vi "CPSControlling.vi"() -> ()   [LabVIEW 2017]
uses:
  classes/DataHandlerMYiTOPS.lvclass
panel:
  in  "Monitoring":T1 {"Meter" scale=0.0..20.0}
  out "appended array":string[](array[string])
  out "element":string
  out "Control-Matrix-Overview 2":i32(listbox)=-1
  in  "Controlling":T2={"LED 1"=FALSE, "Stop Client App"=FALSE, "LED 2"=FALSE, "Drive Motor"=FALSE, "Direcion Moter"=FALSE, "Steps"=512} {"Steps" min=1 step=1}
  in  "Cyber-physical Objects":i32(listbox)
  in  "Stop":bool
  out "Control-Matrix-Overview":i32(listbox)=-1
  # "Hard Key:"
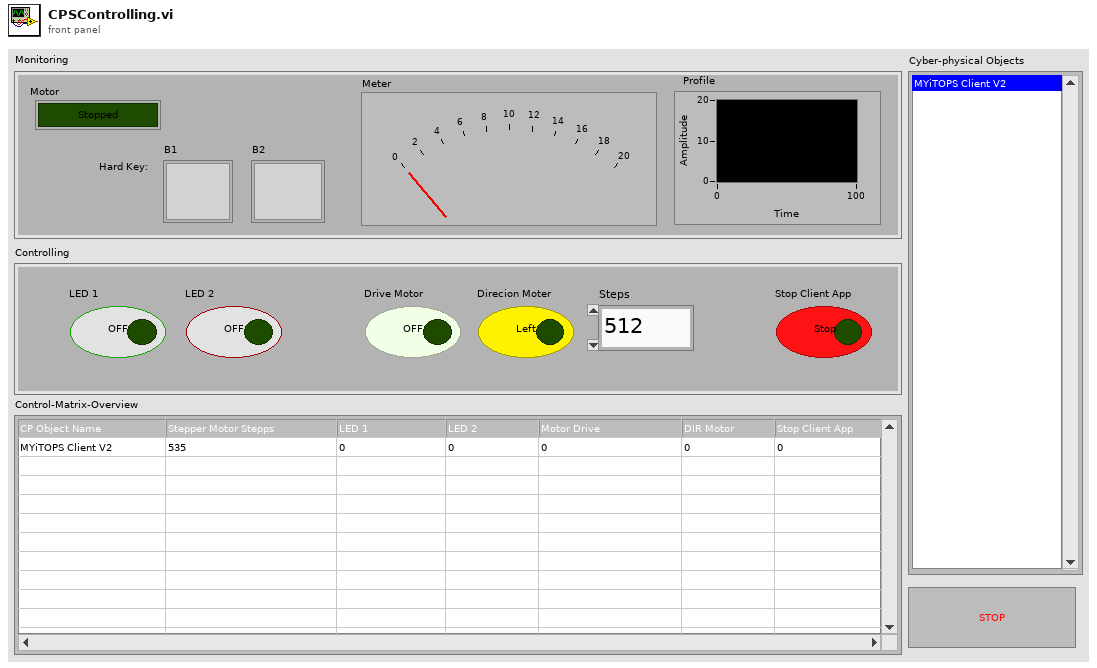
[diagram p1: front panel]
types:
  T1 = cluster{"Meter":i8, "Profile":dbl, "B2":bool, "B1":bool, "Motor":bool}
  T2 = cluster{"LED 1":bool, "Stop Client App":bool, "LED 2":bool, "Drive Motor":bool, "Direcion Moter":bool, "Steps":u64}
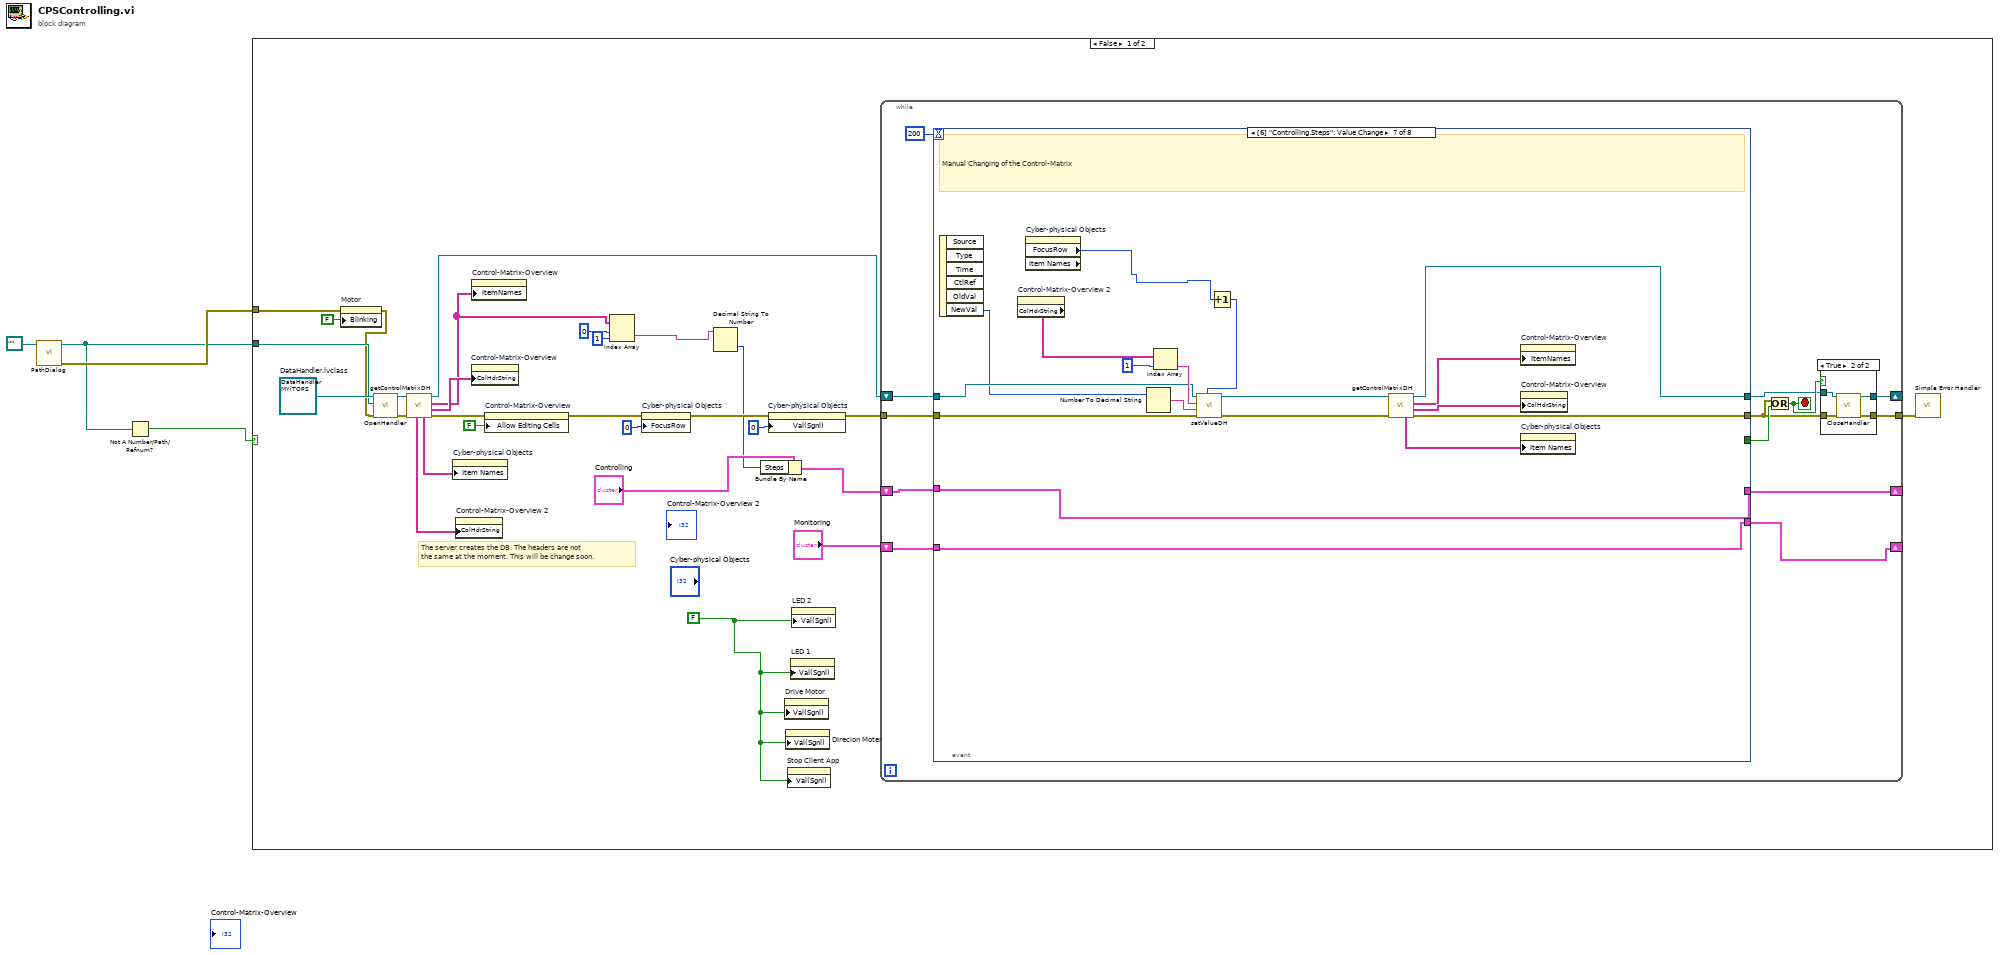
[diagram p0: block diagram]
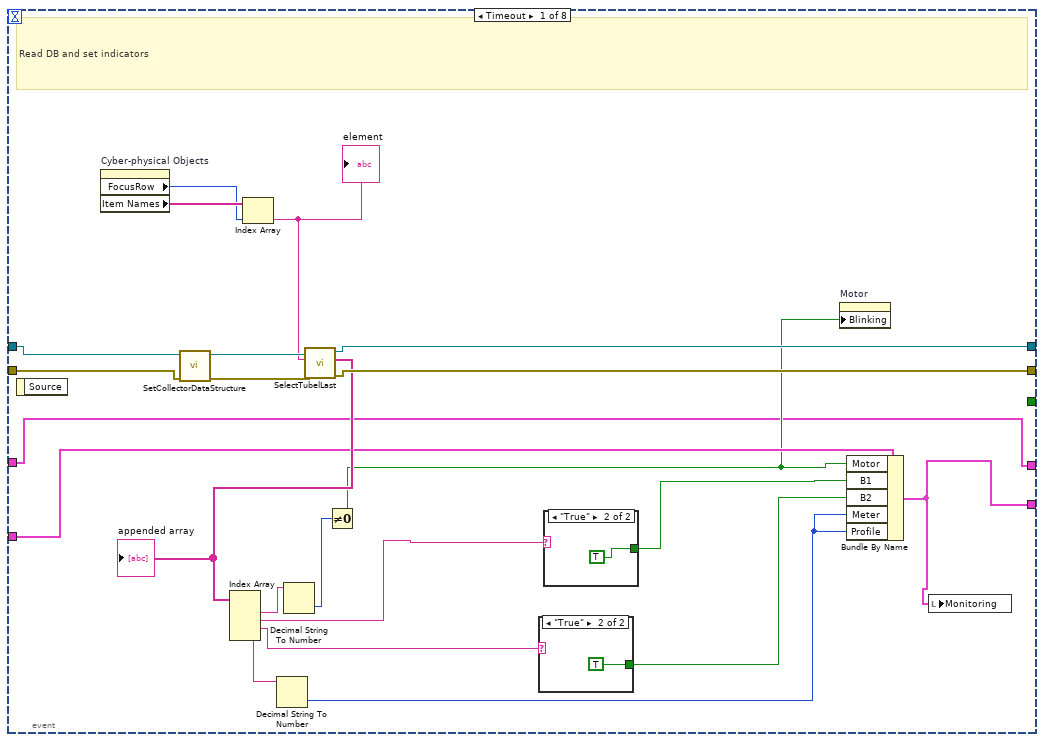
[diagram p3: hidden frame]
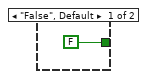
[diagram p4: hidden frame]
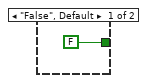
[diagram p5: hidden frame]
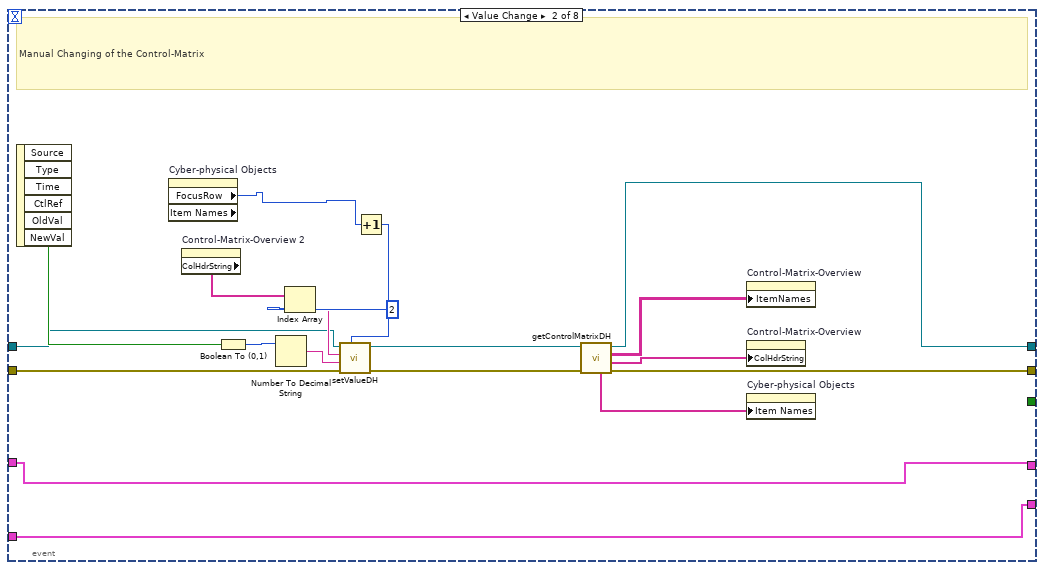
[diagram p6: hidden frame]
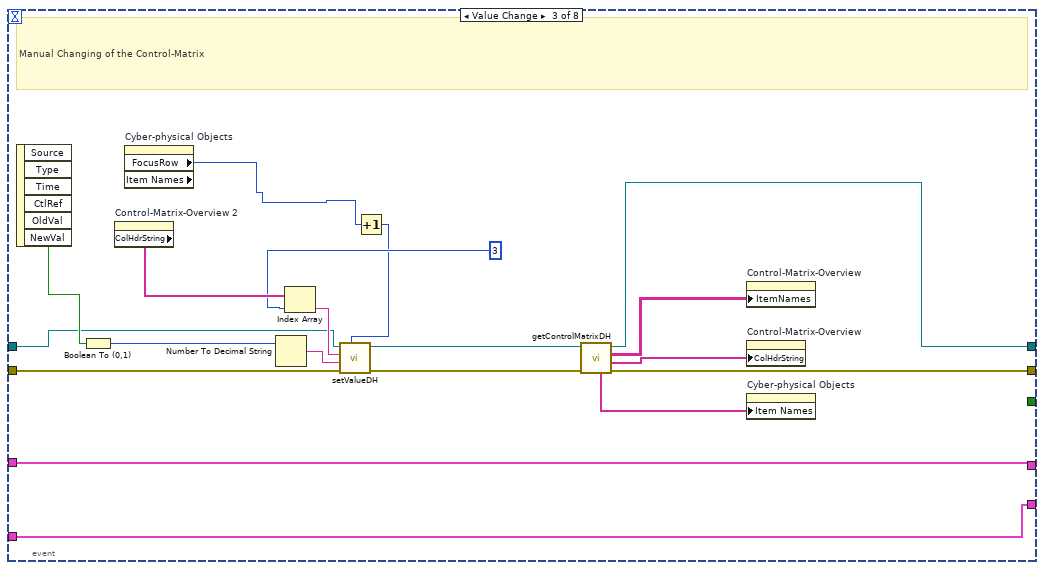
[diagram p7: hidden frame]
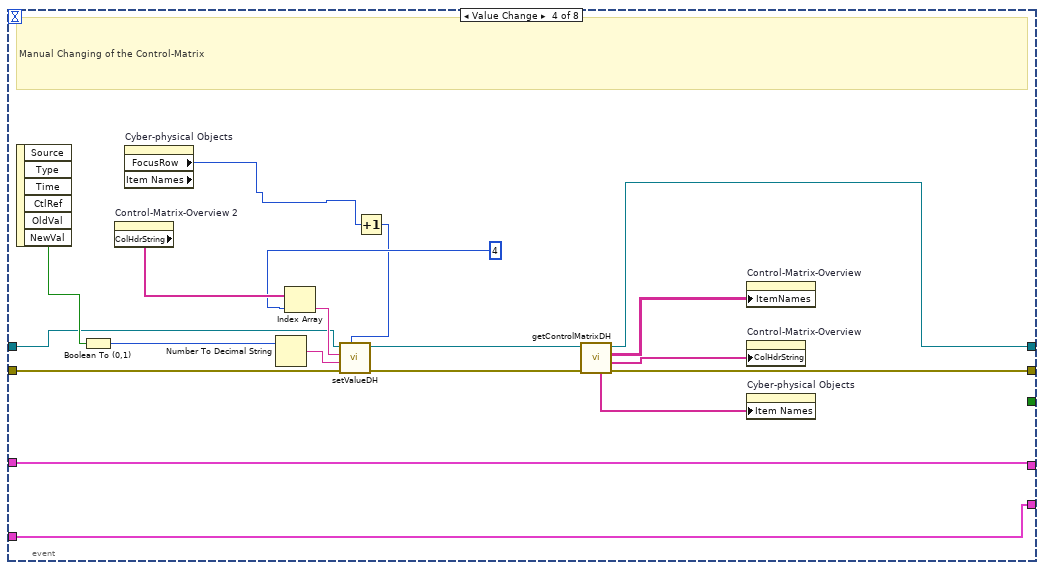
[diagram p8: hidden frame]
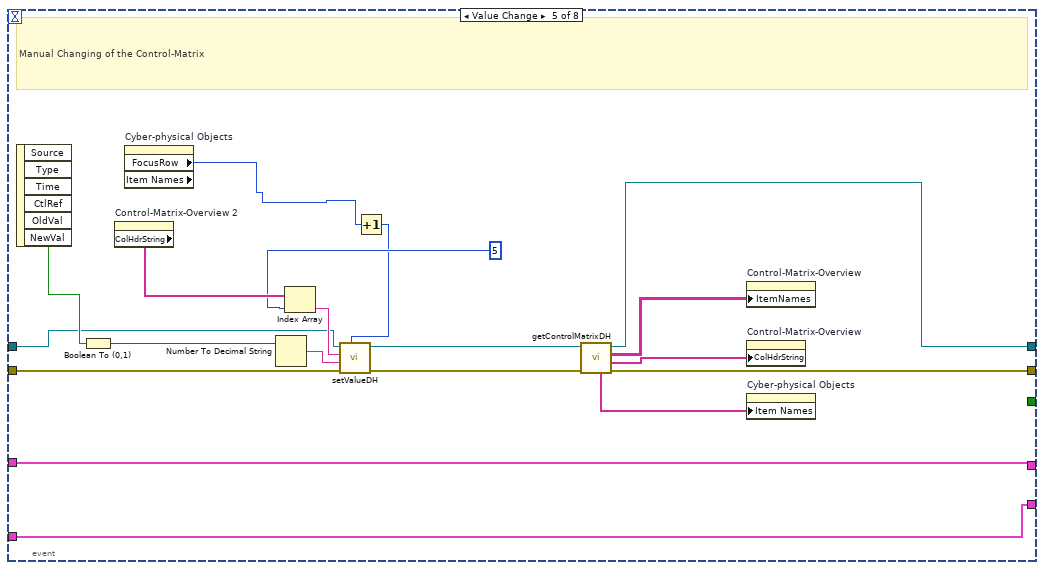
[diagram p9: hidden frame]
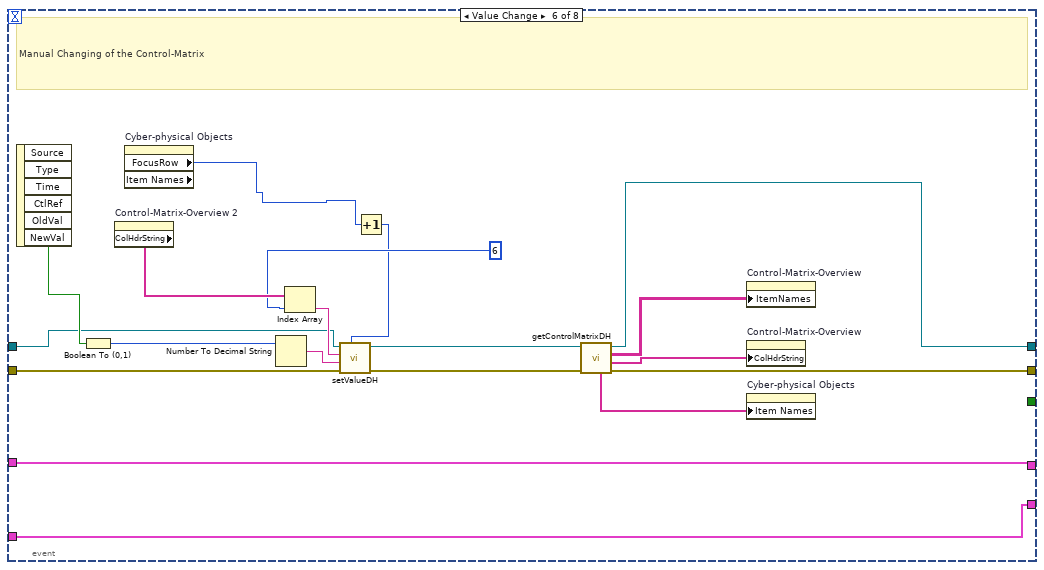
[diagram p10: hidden frame]
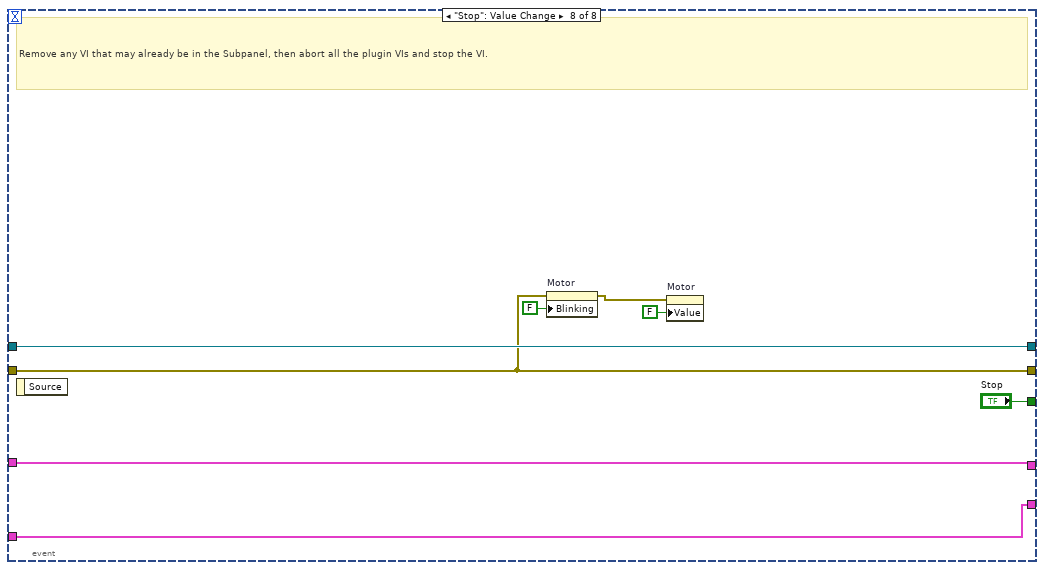
[diagram p11: hidden frame]
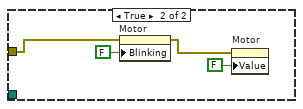
[diagram p12: hidden frame]
diagram:
  n1 = call "PathDialog.vi"("Path to Data Base in"=path "" ("Path to Data Base")) -> ("error out"=w3:errorcluster, "Path to Data Base out"=w2:path)  [unwired: 9 in]
  n2 = Not A Number/Path/Refnum?(number/path/refnum=w2) -> (NaN/Path/Refnum?=w1:bool)
  n3 = case shown="False" w1 {
    tunnel: w2 -> [w17 _]
    tunnel: w3 -> [w14 w201]
    frame False {
      w15 = FALSE ("Value")
      w28 = refnum<class "DataHandlerMYiTOPS.lvclass"> refnum  # DataHandler.lvclass
      # "The server creates the DB. The headers are not \nthe same at the moment. This will be change soon."
      n4 = property on="Motor" class="Bool (strict)"(error in=w14, "Blinking"=FALSE) -> (error out=w13:errorcluster)  [unwired: 1 in, 1 out]
      n5 = call-dynamic "OpenHandler.vi"("error in (no error)"=w13, "path to db monitoring"=w17, "DataHandling in"=w28) -> ("error out"=w27:errorcluster, "DataHandling out"=w26:refnum<class "DataHandlerMYiTOPS.lvclass">)  [unwired: 7 in]
      n6 = call-dynamic "getControlMatrixDH.vi"("error in (no error)"=w27, "DataHandler in"=w26) -> ("error out"=w24:errorcluster, "List of ColHads"=w23:string[], "Array"=w10:string[][], "DataHandler out"=w19:refnum<class "DataHandlerMYiTOPS.lvclass">, "Field Elements"=w25:string[], "List of ColHads 2"=w18:string[])  [unwired: 4 in]
      n7 = property on="Cyber-physical Objects" class="LstBox (strict)"("Item Names"=w25) -> ()  [unwired: 2 in, 2 out]
      n8 = property on="Control-Matrix-Overview 2" class="MCListbox (strict)"("ColHdrString"=w18) -> ()  [unwired: 2 in, 2 out]
      n9 = property on="Control-Matrix-Overview" class="MCListbox (strict)"("ColHdrString"=w23) -> ()  [unwired: 2 in, 2 out]
      n10 = property on="Control-Matrix-Overview" class="MCListbox (strict)"("ItemNames"=w10) -> ()  [unwired: 2 in, 2 out]
      n11 = property on="Control-Matrix-Overview" class="MCListbox (strict)"(error in=w24, "Allow Editing Cells"=FALSE) -> (error out=w20:errorcluster)  [unwired: 1 in, 1 out]
      n12 = Index Array(array=w10, index (row)=0 ("index"), index (col)=1 ("disabled index (col)")) -> (element=w6:string)
      n13 = property on="Cyber-physical Objects" class="LstBox (strict)"(error in=w20, "FocusRow"=0 ("Focus Row")) -> (error out=w21:errorcluster)  [unwired: 1 in, 1 out]
      n14 = Decimal String To Number(string=w6) -> (number=w5:i32)  [unwired: 2 in, 1 out]
      n15 = Bundle By Name(cluster="Controlling", "Steps"=w5) -> (w7:T2)
      n16 = property on="Cyber-physical Objects" class="ListBox (strict)"(error in=w21, "Val(Sgnl)"=u16 0 ("Value (Signaling)")) -> (error out=w32:errorcluster)  [unwired: 1 in, 1 out]
      n17 = property on="Drive Motor" class="Bool (strict)"("Val(Sgnl)"=w15) -> ()  [unwired: 2 in, 2 out]
      n18 = property on="Direcion Moter" class="Bool (strict)"("Val(Sgnl)"=w15) -> ()  [unwired: 2 in, 2 out]
      n19 = property on="Stop Client App" class="Bool (strict)"("Val(Sgnl)"=w15) -> ()  [unwired: 2 in, 2 out]
      n20 = property on="LED 1" class="Bool (strict)"("Val(Sgnl)"=w15) -> ()  [unwired: 2 in, 2 out]
      n21 = property on="LED 2" class="Bool (strict)"("Val(Sgnl)"=w15) -> ()  [unwired: 2 in, 2 out]
      n22 = while {
        tunnel: w32 -> [w44]
        tunnel: [w39] -> w30
        shift-right: [w37] -> _
        shift-left: w19 -> [w42]
        shift-right: [w33] -> _
        shift-left: w7 -> [w36]
        shift-right: [w34] -> _
        shift-left: "Monitoring" -> [w35]
        stop <- w41 stop-if-true
        n23 = event shown="[6] \"Controlling.Steps\": Value Change" {
          selector: _ -> [_ _ _ _ _ _ _ _]
          dyn-events: _ -> [_ _ _ _ _ _ _ _]
          timeout: 200 -> [_ _ _ _ _ _ _ _]
          tunnel: [_ _ _ _ _ _ _ "Stop"] -> w45
          tunnel: [w66 w94 w111 w130 w149 w168 w186 w193] -> w40
          tunnel: w44 -> [w68 w96 w115 w134 w153 w172 w190 w193]
          tunnel: w42 -> [w71 w85 w102 w121 w140 w159 w179 w197]
          tunnel: [w69 w86 w103 w122 w141 w160 w180 w197] -> w38
          tunnel: w36 -> [w52 w82 w98 w117 w136 w155 w173 w196]
          tunnel: [w52 w82 w98 w117 w136 w155 w173 w196] -> w33
          tunnel: w35 -> [w56 w81 w97 w116 w135 w154 w175 w195]
          tunnel: [w55 w81 w97 w116 w135 w154 w175 w195] -> w34
          event Timeout {
            # "Read DB and set indicators"
            n24 = event-data() -> ()  [unwired: 1 in, 1 out]
            n25 = property on="Cyber-physical Objects" class="LstBox (strict)"() -> ("FocusRow"=w72:i32, "Item Names"=w73:string[])  [unwired: 2 in, 2 out]
            n26 = call-dynamic "SetCollectorDataStructure.vi"("error in (no error)"=w68, "DataHandler in"=w71) -> ("error out"=w67:errorcluster, "DataHandler out"=w70:refnum<class "DataHandlerMYiTOPS.lvclass">)  [unwired: 8 in]
            n27 = Index Array(array=w73, index=w72) -> (element=w65:string)
            "element" <- w65
            n28 = call-dynamic "SelectTubelLast.vi"("error in (no error)"=w67, "Unique Object Identifier"=w65, "DataHandler in"=w70) -> ("error out"=w66:errorcluster, "appended array"=w64:string[], "DataHandler out"=w69:refnum<class "DataHandlerMYiTOPS.lvclass">)  [unwired: 6 in]
            "appended array" <- w64
            n29 = Index Array(array=w64) -> (element #1=w63:string, element #2=w62:string, element #3=w61:string, element #4=w60:string)  [unwired: 4 in]
            n30 = Decimal String To Number(string=w60) -> (number=w59:i32)  [unwired: 2 in, 1 out]
            n31 = Decimal String To Number(string=w63) -> (number=w54:i32)  [unwired: 2 in, 1 out]
            n32 = Not Equal To 0?(x=w54) -> (x != 0?=w53:bool)
            n33 = case shown="\"True\"" w61 {
              tunnel: [FALSE TRUE] -> w58
              frame "False", Default {
              }
              frame "True" {
              }
            }
            n34 = case shown="\"True\"" w62 {
              tunnel: [FALSE TRUE] -> w57
              frame "False", Default {
              }
              frame "True" {
              }
            }
            n35 = property on="Motor" class="Bool (strict)"("Blinking"=w53) -> ()  [unwired: 2 in, 2 out]
            n36 = Bundle By Name(cluster=w56, "Motor"=w53, "B1"=w57, "B2"=w58, "Meter"=w59, "Profile"=w59) -> (w55:T1)
            n37 = local write "Monitoring"(w55) -> ()
          }
          event "Controlling.LED 1": Value Change {
            # "Manual Changing of the Control-Matrix"
            n38 = event-data() -> ("NewVal"=w89:bool)  [unwired: 1 in, 5 out]
            n39 = property on="Cyber-physical Objects" class="LstBox (strict)" props=["FocusRow", "Item Names"]() -> ("FocusRow"=w84:i32)  [unwired: 2 in, 3 out]
            n40 = property on="Control-Matrix-Overview 2" class="MCListbox (strict)"() -> ("ColHdrString"=w92:string[])  [unwired: 2 in, 2 out]
            n41 = Boolean To (0,1)(Boolean=w89) -> (0, 1=w88:i16)
            n42 = Number To Decimal String(number=w88) -> (decimal integer string=w93:string)  [unwired: 1 in]
            n43 = Index Array(array=w92, index=2) -> (element=w90:string)
            n44 = Increment(x=w84) -> (x+1=w83:i32)
            n45 = call-dynamic "setValueDH.vi"("Focus"=w83, "error in (no error)"=w96, "Value"=w93, "ItemName"=w90, "DataHandler in"=w85) -> ("error out"=w95:errorcluster, "DataHandler out"=w87:refnum<class "DataHandlerMYiTOPS.lvclass">)  [unwired: 5 in]
            n46 = call-dynamic "getControlMatrixDH.vi"("error in (no error)"=w95, "DataHandler in"=w87) -> ("error out"=w94:errorcluster, "List of ColHads"=w79:string[], "Array"=w78:string[][], "DataHandler out"=w86:refnum<class "DataHandlerMYiTOPS.lvclass">, "Field Elements"=w80:string[])  [unwired: 4 in, 1 out]
            n47 = property on="Control-Matrix-Overview" class="MCListbox (strict)"("ItemNames"=w78) -> ()  [unwired: 2 in, 2 out]
            n48 = property on="Control-Matrix-Overview" class="MCListbox (strict)"("ColHdrString"=w79) -> ()  [unwired: 2 in, 2 out]
            n49 = property on="Cyber-physical Objects" class="LstBox (strict)"("Item Names"=w80) -> ()  [unwired: 2 in, 2 out]
          }
          event "Controlling.LED 2": Value Change {
            # "Manual Changing of the Control-Matrix"
            n50 = event-data() -> ("NewVal"=w106:bool)  [unwired: 1 in, 5 out]
            n51 = Boolean To (0,1)(Boolean=w106) -> (0, 1=w105:i16)
            n52 = property on="Control-Matrix-Overview 2" class="MCListbox (strict)"() -> ("ColHdrString"=w109:string[])  [unwired: 2 in, 2 out]
            n53 = property on="Cyber-physical Objects" class="LstBox (strict)" props=["FocusRow", "Item Names"]() -> ("FocusRow"=w100:i32)  [unwired: 2 in, 3 out]
            n54 = Number To Decimal String(number=w105) -> (decimal integer string=w110:string)  [unwired: 1 in]
            n55 = Index Array(array=w109, index=3) -> (element=w107:string)
            n56 = Increment(x=w100) -> (x+1=w99:i32)
            n57 = call-dynamic "setValueDH.vi"("Focus"=w99, "error in (no error)"=w115, "Value"=w110, "ItemName"=w107, "DataHandler in"=w102) -> ("error out"=w112:errorcluster, "DataHandler out"=w104:refnum<class "DataHandlerMYiTOPS.lvclass">)  [unwired: 5 in]
            n58 = call-dynamic "getControlMatrixDH.vi"("error in (no error)"=w112, "DataHandler in"=w104) -> ("error out"=w111:errorcluster, "List of ColHads"=w113:string[], "Array"=w101:string[][], "DataHandler out"=w103:refnum<class "DataHandlerMYiTOPS.lvclass">, "Field Elements"=w114:string[])  [unwired: 4 in, 1 out]
            n59 = property on="Control-Matrix-Overview" class="MCListbox (strict)"("ItemNames"=w101) -> ()  [unwired: 2 in, 2 out]
            n60 = property on="Control-Matrix-Overview" class="MCListbox (strict)"("ColHdrString"=w113) -> ()  [unwired: 2 in, 2 out]
            n61 = property on="Cyber-physical Objects" class="LstBox (strict)"("Item Names"=w114) -> ()  [unwired: 2 in, 2 out]
          }
          event "Controlling.Drive Motor": Value Change {
            # "Manual Changing of the Control-Matrix"
            n62 = event-data() -> ("NewVal"=w125:bool)  [unwired: 1 in, 5 out]
            n63 = Boolean To (0,1)(Boolean=w125) -> (0, 1=w124:i16)
            n64 = property on="Control-Matrix-Overview 2" class="MCListbox (strict)"() -> ("ColHdrString"=w128:string[])  [unwired: 2 in, 2 out]
            n65 = property on="Cyber-physical Objects" class="LstBox (strict)" props=["FocusRow", "Item Names"]() -> ("FocusRow"=w119:i32)  [unwired: 2 in, 3 out]
            n66 = Number To Decimal String(number=w124) -> (decimal integer string=w129:string)  [unwired: 1 in]
            n67 = Index Array(array=w128, index=4) -> (element=w126:string)
            n68 = Increment(x=w119) -> (x+1=w118:i32)
            n69 = call-dynamic "setValueDH.vi"("Focus"=w118, "error in (no error)"=w134, "Value"=w129, "ItemName"=w126, "DataHandler in"=w121) -> ("error out"=w131:errorcluster, "DataHandler out"=w123:refnum<class "DataHandlerMYiTOPS.lvclass">)  [unwired: 5 in]
            n70 = call-dynamic "getControlMatrixDH.vi"("error in (no error)"=w131, "DataHandler in"=w123) -> ("error out"=w130:errorcluster, "List of ColHads"=w132:string[], "Array"=w120:string[][], "DataHandler out"=w122:refnum<class "DataHandlerMYiTOPS.lvclass">, "Field Elements"=w133:string[])  [unwired: 4 in, 1 out]
            n71 = property on="Control-Matrix-Overview" class="MCListbox (strict)"("ItemNames"=w120) -> ()  [unwired: 2 in, 2 out]
            n72 = property on="Control-Matrix-Overview" class="MCListbox (strict)"("ColHdrString"=w132) -> ()  [unwired: 2 in, 2 out]
            n73 = property on="Cyber-physical Objects" class="LstBox (strict)"("Item Names"=w133) -> ()  [unwired: 2 in, 2 out]
          }
          event "Controlling.Direcion Moter": Value Change {
            # "Manual Changing of the Control-Matrix"
            n74 = event-data() -> ("NewVal"=w144:bool)  [unwired: 1 in, 5 out]
            n75 = Boolean To (0,1)(Boolean=w144) -> (0, 1=w143:i16)
            n76 = property on="Control-Matrix-Overview 2" class="MCListbox (strict)"() -> ("ColHdrString"=w147:string[])  [unwired: 2 in, 2 out]
            n77 = property on="Cyber-physical Objects" class="LstBox (strict)" props=["FocusRow", "Item Names"]() -> ("FocusRow"=w138:i32)  [unwired: 2 in, 3 out]
            n78 = Number To Decimal String(number=w143) -> (decimal integer string=w148:string)  [unwired: 1 in]
            n79 = Index Array(array=w147, index=5) -> (element=w145:string)
            n80 = Increment(x=w138) -> (x+1=w137:i32)
            n81 = call-dynamic "setValueDH.vi"("Focus"=w137, "error in (no error)"=w153, "Value"=w148, "ItemName"=w145, "DataHandler in"=w140) -> ("error out"=w150:errorcluster, "DataHandler out"=w142:refnum<class "DataHandlerMYiTOPS.lvclass">)  [unwired: 5 in]
            n82 = call-dynamic "getControlMatrixDH.vi"("error in (no error)"=w150, "DataHandler in"=w142) -> ("error out"=w149:errorcluster, "List of ColHads"=w151:string[], "Array"=w139:string[][], "DataHandler out"=w141:refnum<class "DataHandlerMYiTOPS.lvclass">, "Field Elements"=w152:string[])  [unwired: 4 in, 1 out]
            n83 = property on="Control-Matrix-Overview" class="MCListbox (strict)"("ItemNames"=w139) -> ()  [unwired: 2 in, 2 out]
            n84 = property on="Control-Matrix-Overview" class="MCListbox (strict)"("ColHdrString"=w151) -> ()  [unwired: 2 in, 2 out]
            n85 = property on="Cyber-physical Objects" class="LstBox (strict)"("Item Names"=w152) -> ()  [unwired: 2 in, 2 out]
          }
          event "Controlling.Stop Client App": Value Change {
            # "Manual Changing of the Control-Matrix"
            n86 = event-data() -> ("NewVal"=w163:bool)  [unwired: 1 in, 5 out]
            n87 = Boolean To (0,1)(Boolean=w163) -> (0, 1=w162:i16)
            n88 = property on="Control-Matrix-Overview 2" class="MCListbox (strict)"() -> ("ColHdrString"=w166:string[])  [unwired: 2 in, 2 out]
            n89 = property on="Cyber-physical Objects" class="LstBox (strict)" props=["FocusRow", "Item Names"]() -> ("FocusRow"=w157:i32)  [unwired: 2 in, 3 out]
            n90 = Number To Decimal String(number=w162) -> (decimal integer string=w167:string)  [unwired: 1 in]
            n91 = Index Array(array=w166, index=6) -> (element=w164:string)
            n92 = Increment(x=w157) -> (x+1=w156:i32)
            n93 = call-dynamic "setValueDH.vi"("Focus"=w156, "error in (no error)"=w172, "Value"=w167, "ItemName"=w164, "DataHandler in"=w159) -> ("error out"=w169:errorcluster, "DataHandler out"=w161:refnum<class "DataHandlerMYiTOPS.lvclass">)  [unwired: 5 in]
            n94 = call-dynamic "getControlMatrixDH.vi"("error in (no error)"=w169, "DataHandler in"=w161) -> ("error out"=w168:errorcluster, "List of ColHads"=w170:string[], "Array"=w158:string[][], "DataHandler out"=w160:refnum<class "DataHandlerMYiTOPS.lvclass">, "Field Elements"=w171:string[])  [unwired: 4 in, 1 out]
            n95 = property on="Control-Matrix-Overview" class="MCListbox (strict)"("ItemNames"=w158) -> ()  [unwired: 2 in, 2 out]
            n96 = property on="Control-Matrix-Overview" class="MCListbox (strict)"("ColHdrString"=w170) -> ()  [unwired: 2 in, 2 out]
            n97 = property on="Cyber-physical Objects" class="LstBox (strict)"("Item Names"=w171) -> ()  [unwired: 2 in, 2 out]
          }
          event "Controlling.Steps": Value Change {
            # "Manual Changing of the Control-Matrix"
            n98 = event-data() -> ("NewVal"=w174:u64)  [unwired: 1 in, 5 out]
            n99 = property on="Control-Matrix-Overview 2" class="MCListbox (strict)"() -> ("ColHdrString"=w184:string[])  [unwired: 2 in, 2 out]
            n100 = property on="Cyber-physical Objects" class="LstBox (strict)" props=["FocusRow", "Item Names"]() -> ("FocusRow"=w177:i32)  [unwired: 2 in, 3 out]
            n101 = Number To Decimal String(number=w174) -> (decimal integer string=w185:string)  [unwired: 1 in]
            n102 = Index Array(array=w184, index=1) -> (element=w182:string)
            n103 = Increment(x=w177) -> (x+1=w176:i32)
            n104 = call-dynamic "setValueDH.vi"("Focus"=w176, "error in (no error)"=w190, "Value"=w185, "ItemName"=w182, "DataHandler in"=w179) -> ("error out"=w187:errorcluster, "DataHandler out"=w181:refnum<class "DataHandlerMYiTOPS.lvclass">)  [unwired: 5 in]
            n105 = call-dynamic "getControlMatrixDH.vi"("error in (no error)"=w187, "DataHandler in"=w181) -> ("error out"=w186:errorcluster, "List of ColHads"=w188:string[], "Array"=w178:string[][], "DataHandler out"=w180:refnum<class "DataHandlerMYiTOPS.lvclass">, "Field Elements"=w189:string[])  [unwired: 4 in, 1 out]
            n106 = property on="Control-Matrix-Overview" class="MCListbox (strict)"("ItemNames"=w178) -> ()  [unwired: 2 in, 2 out]
            n107 = property on="Control-Matrix-Overview" class="MCListbox (strict)"("ColHdrString"=w188) -> ()  [unwired: 2 in, 2 out]
            n108 = property on="Cyber-physical Objects" class="LstBox (strict)"("Item Names"=w189) -> ()  [unwired: 2 in, 2 out]
          }
          event "Stop": Value Change {
            # "Remove any VI that may already be in the Subpanel, then abort all the plugin VIs and stop the VI."
            n109 = event-data() -> ()  [unwired: 1 in, 1 out]
            n110 = property on="Motor" class="Bool (strict)"(error in=w193, "Blinking"=FALSE) -> (error out=w192:errorcluster)  [unwired: 1 in, 1 out]
            n111 = property on="Motor" class="Bool (strict)"(error in=w192, "Value"=FALSE) -> ()  [unwired: 1 in, 2 out]
          }
        }
        n112 = Or(x=w40, y=w45) -> (x .or. y?=w41:bool)
        n113 = case shown="True" w41 {
          tunnel: w40 -> [w47 w50]
          tunnel: [w47 w51] -> w39
          tunnel: w38 -> [w46 w49]
          tunnel: [w46 w48] -> w37
          frame False {
          }
          frame True {
            n114 = call-dynamic "CloseHandler.vi"("error in (no error)"=w50, "DataHandling in"=w49) -> ("error out"=w51:errorcluster, "DataHandling out"=w48:refnum<class "DataHandlerMYiTOPS.lvclass">)  [unwired: 8 in]
          }
        }
      }
      n115 = call <vilib>:"Simple Error Handler.vi"("error in (no error)"=w30) -> ()  [unwired: 4 in, 5 out]
    }
    frame True {
      n116 = property on="Motor" class="Bool (strict)"(error in=w201, "Blinking"=FALSE) -> (error out=w199:errorcluster)  [unwired: 1 in, 1 out]
      n117 = property on="Motor" class="Bool (strict)"(error in=w199, "Value"=FALSE) -> ()  [unwired: 1 in, 2 out]
    }
  }
